vi "Write--init.vi"(8 "error in (no error)":errorcluster, 10 "Comando":T1 {"Action" items=["Initialize", "Move"]}, 11 "VISA resource name":refnum<visa-resource-name>) -> (0 "error out":errorcluster, 2 "Comando(string)":string, 3 "VISA resource name out":refnum<visa-resource-name>)   [LabVIEW 2020, in "Control de MaP.lvlib"]
doc: "convierte la selección de comando a cadena y lo envía al puerto seleccionado"
uses:
  Control de MaP.lvlib
  <vilib>/Instr/_visa.llb/VISA Flush IO Buffer Mask.ctl
  Controls/Motor initialization parameters--cluster.ctl
panel:
  out "return count":u32
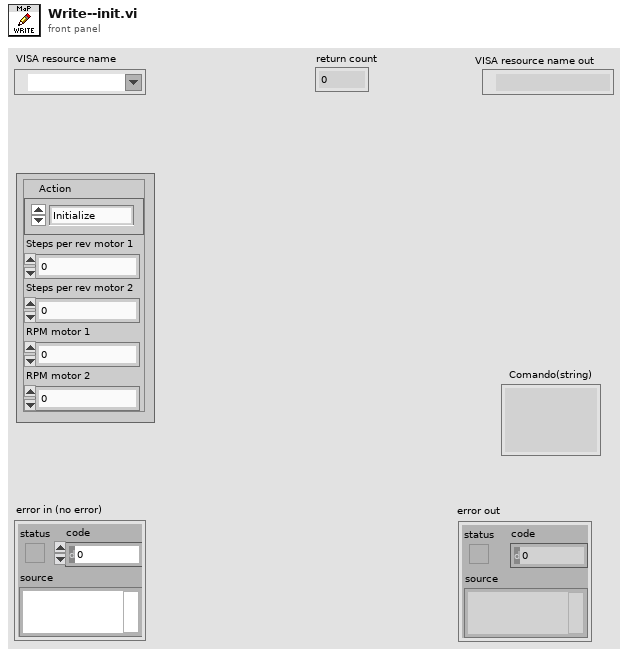
[diagram p1: front panel]
types:
  T1 = typedef "Control de MaP.lvlib/Motor initialization parameters--cluster.ctl" = cluster{"Action":u8, "Steps per rev motor 1":u8, "Steps per rev motor 2":u8, "RPM motor 1":u16, "RPM motor 2":u16}
  T2 = typedef "VISA Flush IO Buffer Mask.ctl" = u16
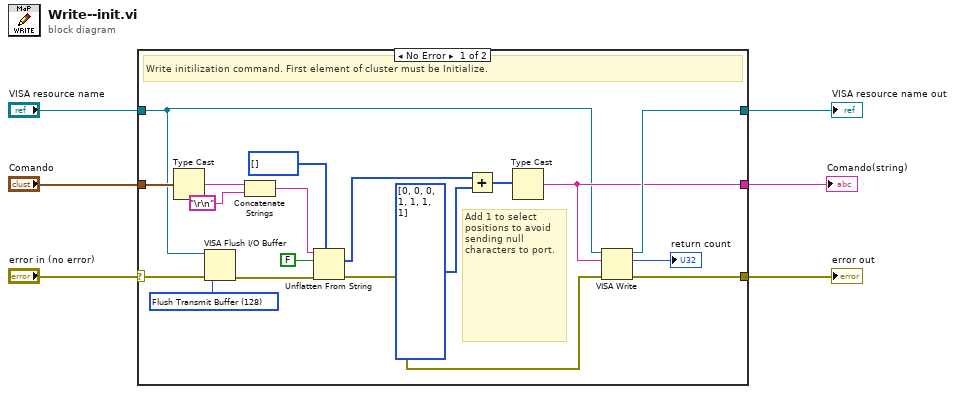
[diagram p0: block diagram]
diagram:
  n1 = case shown="No Error" "error in (no error)" {
    selector: "error in (no error)" -> [w13 w26]
    tunnel: "VISA resource name" -> [w11 w25]
    tunnel: [w24 w25] -> w5
    tunnel: [w23 w26] -> w3
    tunnel: "Comando" -> [w22 _]
    tunnel: [w14 _] -> w1
    frame No Error {
      w10 = T2 128 items=["Flush Receive Buffer"=16, "Write Transmit Buffer to Device"=32, "Flush Receive Buffer (No I/O)"=64, "Flush Transmit Buffer"=128] ("Mask")
      # "Add 1 to select positions to avoid sending null characters to port."
      # "Write initilization command. First element of cluster must be Initialize."
      n2 = Type Cast(x=w22) -> (*(type *) &x=w9:string)  [unwired: 1 in]
      n3 = VISA Flush I/O Buffer(VISA resource name=w11, mask (16)=w10, error in (no error)=w13) -> (error out=w12:errorcluster)  [unwired: 1 out]
      n4 = Concatenate Strings(w9, "\r\n") -> (w8:string)
      n5 = Unflatten From String(type=u8[] [], binary string=w8, data includes array or string size? (T)=FALSE, error in (no error)=w12) -> (value=w15:u8[], error out=w16:errorcluster)  [unwired: 1 in, 1 out]
      n6 = Add(x=w15, y=u8[] [0, 0, 0, 1, 1, 1, 1]) -> (x+y=w17:u8[])
      n7 = Type Cast(x=w17) -> (*(type *) &x=w14:string)  [unwired: 1 in]
      n8 = VISA Write(VISA resource name=w11, write buffer=w14, error in (no error)=w16) -> (VISA resource name out=w24:refnum<visa-resource-name>, return count=→"return count":u32, error out=w23:errorcluster)
    }
    frame Error {
    }
  }
  "VISA resource name out" <- w5
  "error out" <- w3
  "Comando(string)" <- w1
